vi "Nod_Head.vi"(0 "error in":errorcluster, 3 "node":string) -> (1 "error out":errorcluster)   [LabVIEW 2010]
doc: "This will nod the head."
uses:
  <userlib>/ROSforLV_0.1/ROS/MessageBuilding/Primitives/subs/boolScalar.vi
panel:
  in  "State":bool=TRUE
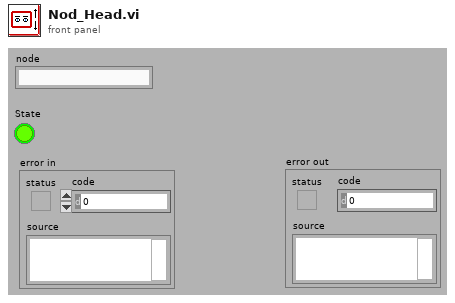
[diagram p1: front panel]
types:
  T1 = typedef "_ROSControl.ctl" = cluster{"topic port":u16, "Node":string, "topic":string, "type":string, "node port":u32, "error ":errorcluster, "Direction":T2, "APIs":string[]}
  T2 = typedef "_ROSDirection.ctl" = enum16{"Node", "Publisher", "Subscriber", "Service Client"}
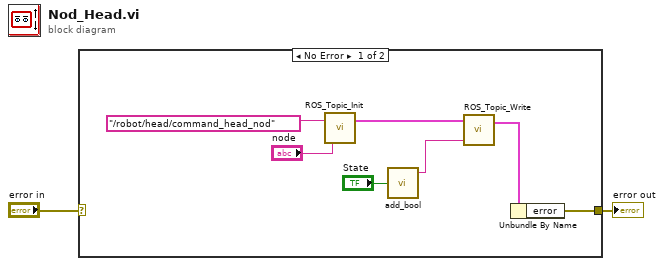
[diagram p0: block diagram]
diagram:
  n1 = case shown="No Error" "error in" {
    selector: "error in" -> [_ w10]
    tunnel: [w6 w10] -> w2
    frame No Error {
      n2 = call <userlib>:"ROS_Topic_Init.vi"("node"="node", "topic"="/robot/head/command_head_nod") -> ("ROS out"=w8:T1)  [unwired: 1 in]
      n3 = call-poly <userlib>:"add_bool.vi"("Boolean"="State") -> ("msg out"=w4:string)  [unwired: 4 in]
      n4 = call <userlib>:"ROS_Topic_Write.vi"("Msg in"=w4, "ROS in"=w8) -> ("ROS out"=w7:T1)  [unwired: 2 in]
      n5 = Unbundle By Name(w7) -> ("error"=w6:errorcluster)
    }
    frame Error {
    }
  }
  "error out" <- w2
